vi "test_Write Bool Register Value.vi"(8 "error in (no error)":errorcluster, 11 "TestCase in":refnum<class "FPGA Register IO Tests.lvclass">=refnum) -> (0 "error out":errorcluster, 3 "TestCase out":refnum<class "FPGA Register IO Tests.lvclass">)   [LabVIEW 2026, in "FPGA Register IO Tests.lvclass"]
uses:
  FPGA Register IO Tests.lvclass
  FPGA Register IO Tests.lvclass/FPGA Register IO Tests.ctl
  APIs/FPGA Register IO/FPGA Register IO.lvlib
  <vilib>/rvi/interface/nirviCloseFPGA/nirviCloseFPGA.xnode
  <vilib>/FPGAPlugInAG/Dynamic/niLvFpga_Close_Dynamic.vi
  Addon/Addon Engine/FPGA Addon Engine.lvlib
  APIs/FPGA Register IO/Write Methods/Write Data Register/Instances/Write Boolean.vi
  APIs/FPGA Register IO/Read Methods/Read Data Register/Instances/Read Boolean.vi
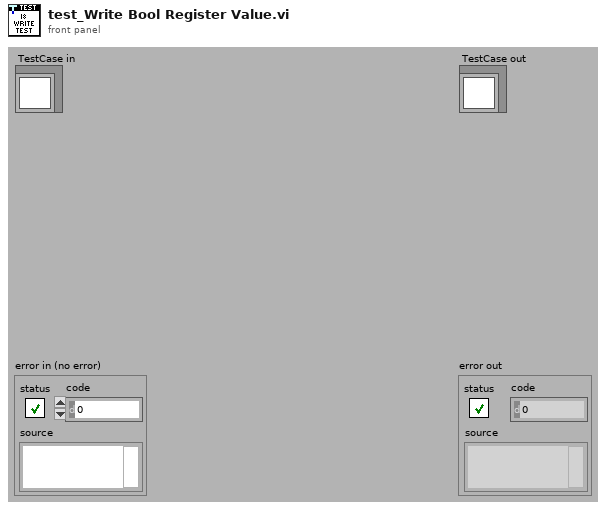
[diagram p1: front panel]
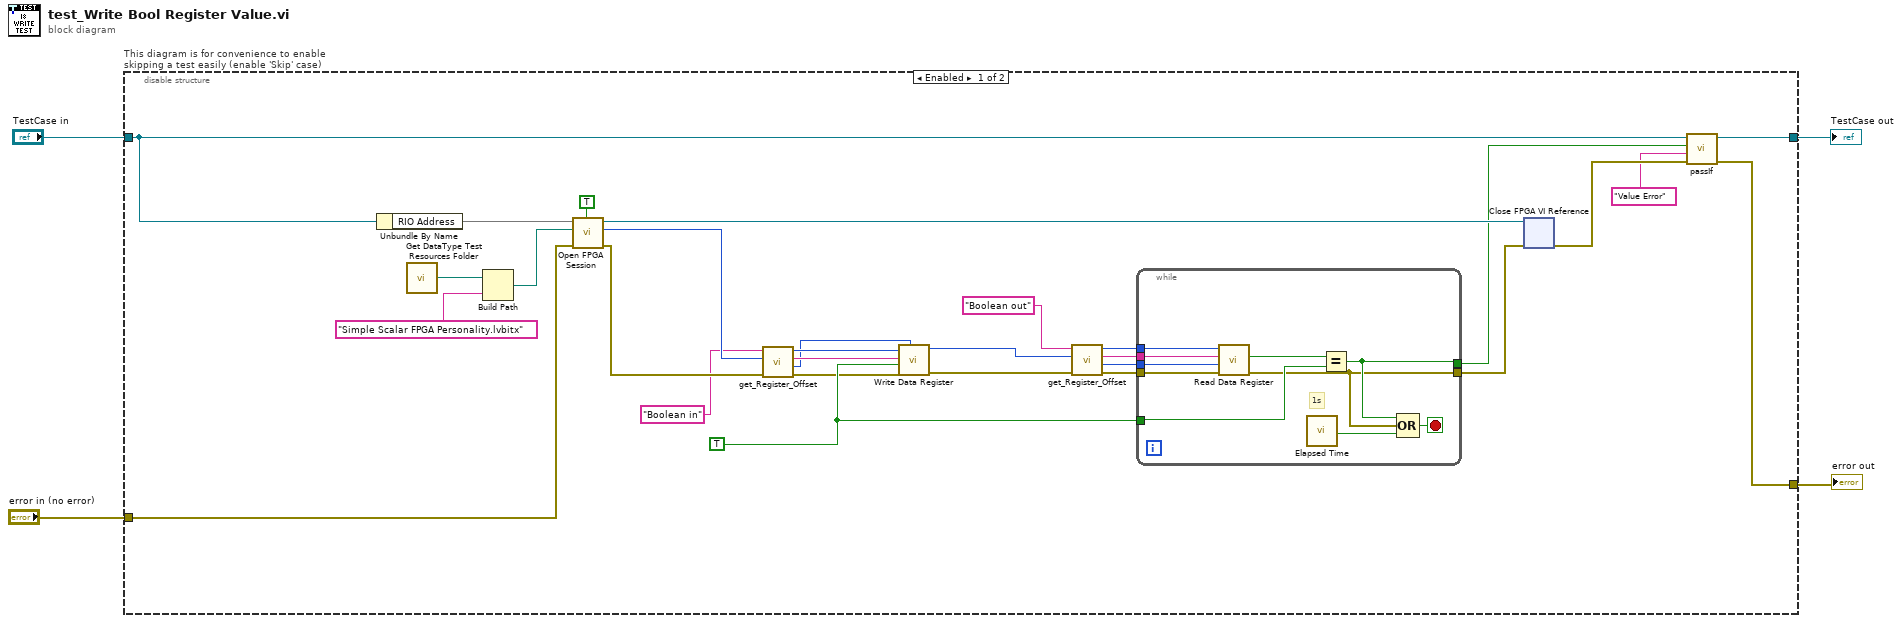
[diagram p0: block diagram]
diagram:
  n1 = disable-structure "This diagram is for convenience to enable skipping a test easily (enable 'Skip' case)" shown="Enabled" {
    disable-tunnel: "TestCase in" -> [w22 w47]
    disable-tunnel: [w25 w45] -> w1
    disable-tunnel: [w24 w46] -> w3
    disable-tunnel: "error in (no error)" -> [w29 w44]
    frame Enabled {
      w17 = TRUE ("value in")
      n2 = Unbundle By Name(w22) -> ("RIO Address"=w23)
      n3 = call "Get DataType Test Resources Folder.vi"() -> ("path"=w27:path)
      n4 = Build Path(base path=w27, name or relative path="Simple Scalar FPGA Personality.lvbitx") -> (appended path=w30:path)
      n5 = call "Open FPGA Session.vi"("run when loaded (T)"=TRUE ("Run When Loaded (T)"), "error in"=w29, "bitfile path"=w30, "device address"=w23) -> ("error out"=w21:errorcluster, "session out"=w15:u32, "bitfile reference out"=w32:refnum<k20>)  [unwired: 5 in]
      n6 = call "get_Register_Offset.vi"("error in (no error)"=w21, "session"=w15, "Name"="Boolean in" ("register name")) -> ("error out"=w16:errorcluster, "RegisterOffset"=w11:u32, "Register Name"=w12:string, "session out"=w14:u32)  [unwired: 5 in]
      n7 = call-poly "Write Data Register.vi"("RegisterOffset"=w11, "error in"=w16, "value in"=w17, "register name"=w12, "session in"=w14) -> ("error out"=w20:errorcluster, "session out"=w9:u32)  [unwired: 5 in]
      n8 = call "get_Register_Offset.vi"("error in (no error)"=w20, "session"=w9, "Name"="Boolean out" ("registerName")) -> ("error out"=w10:errorcluster, "RegisterOffset"=w5:u32, "Register Name"=w7:string, "session out"=w8:u32)  [unwired: 5 in]
      n9 = while {
        tunnel: [w37] -> w19
        tunnel: w10 -> [w43]
        tunnel: w8 -> [w42]
        tunnel: w17 -> [w41]
        tunnel: [w38] -> w18
        tunnel: w7 -> [w35]
        tunnel: w5 -> [w34]
        stop <- w39 stop-if-true
        # "1s"
        n10 = call-poly "Read Data Register.vi"("error in"=w43, "RegisterOffset"=w34, "register name"=w35, "session in"=w42) -> ("error out"=w37:errorcluster, "value out"=w40:bool)  [unwired: 5 in, 1 out]
        n11 = call "Elapsed Time"() -> ("Time has Elapsed"=w36:bool)  [unwired: 12 in, 7 out]
        n12 = Equal?(x=w40, y=w41) -> (x = y?=w38:bool)
        n13 = Compound Arithmetic op=OR(w38, w37, w36) -> (w39:bool)
      }
      n14 = xnode "Close FPGA VI Reference"("FPGA VI Reference In"=w32, "error in"=w19) -> ("error out"=w28:errorcluster)
      n15 = call-dynamic "passIf.vi"("error in (no error)"=w28, "message (\"\")"="Value Error" ("message (\"\")"), "pass"=w18, "TestCase in"=w22) -> ("error out"=w24:errorcluster, "TestCase out"=w25:refnum<class "FPGA Register IO Tests.lvclass">)  [unwired: 6 in]
    }
    frame Disabled {
      # "skip test result while test is under development"
      n16 = call <vilib>:"skip.vi"("error in (no error)"=w44, "TestCase in"=w47) -> ("error out"=w46:errorcluster, "TestCase out"=w45:refnum<class "FPGA Register IO Tests.lvclass">)  [unwired: 8 in]
    }
  }
  "error out" <- w3
  "TestCase out" <- w1
